vi "input.vi"(8 "error in":errorcluster, 10 "data table in":T1, 11 "JSON_RPC_Interface runtime in":refnum<class "JSON_RPC_Interface runtime.lvclass">) -> (0 "error out":errorcluster, 2 "data table out":T1, 3 "JSON_RPC_Interface runtime out":refnum<class "JSON_RPC_Interface runtime.lvclass">)   [LabVIEW 2017, in "JSON_RPC_Interface runtime.lvclass"]
doc: "Provides an interface for reading data from a module at runtime. While this interface performs no operations, a child should provide an override which may read from any open sessions, references, or interfaces."
uses:
  JSON_RPC_Interface runtime.lvclass
  <vilib>/NI/Tag Bus/table/data table.ctl
  JSON_RPC_Interface runtime.lvclass/JSON_RPC_Interface runtime.ctl
  <vilib>/NI/NI JSONRPC Server Framework/Classes/Request/Request.lvclass/Request.ctl
  <vilib>/NI/Tag Bus/table/data polymorphs/write one/write Double.vi
  <vilib>/NI/Tag Bus/table/data polymorphs/write one/write Single.vi
  <vilib>/NI/Tag Bus/table/data polymorphs/write one/write I64.vi
  <vilib>/NI/Tag Bus/table/data polymorphs/write one/write I32.vi
  <vilib>/NI/Tag Bus/table/data polymorphs/write one/write I16.vi
  <vilib>/NI/Tag Bus/table/data polymorphs/write one/write I8.vi
  <vilib>/NI/Tag Bus/table/data polymorphs/write one/write U64.vi
  <vilib>/NI/Tag Bus/table/data polymorphs/write one/write U32.vi
  <vilib>/NI/Tag Bus/table/data polymorphs/write one/write U16.vi
  <vilib>/NI/Tag Bus/table/data polymorphs/write one/write U8.vi
  <vilib>/NI/Tag Bus/table/data polymorphs/write one/write Array of Double.vi
  <vilib>/NI/Tag Bus/table/data polymorphs/write one/write Array of Single.vi
  <vilib>/NI/Tag Bus/table/data polymorphs/write one/write Array of I32.vi
  <vilib>/NI/Tag Bus/table/data polymorphs/write one/write Array of I16.vi
  <vilib>/NI/Tag Bus/table/data polymorphs/write one/write Array of I8.vi
  <vilib>/NI/Tag Bus/table/data polymorphs/write one/write Array of U64.vi
  <vilib>/NI/Tag Bus/table/data polymorphs/write one/write Array of U32.vi
  <vilib>/NI/Tag Bus/table/data polymorphs/write one/write Array of U16.vi
  <vilib>/NI/Tag Bus/table/data polymorphs/write one/write Array of U8.vi
  <vilib>/NI/Tag Bus/table/data polymorphs/write one/write Array of Boolean.vi
  <vilib>/NI/Tag Bus/table/data polymorphs/write one/write Array of String.vi
  <vilib>/NI/Tag Bus/table/data polymorphs/write one/write Boolean.vi
  <vilib>/NI/Tag Bus/table/data polymorphs/write one/write String.vi
  <vilib>/NI/NI JSONRPC Server Framework/Classes/Request/request.Read params.vi
  <vilib>/NI/NI JSONRPC Server Framework/Classes/Request/request.Read method.vi
  <vilib>/NI/JSON Support for LabVIEW/JSON Value/New JSON Value/New JSON ({String}).vi
  <vilib>/NI/NI JSONRPC Server Framework/Classes/Server/Add Response (Method Not Found from Request).vi
  <vilib>/NI/NI JSONRPC Server Framework/Classes/params/params.To JSON Tree.vi
  <vilib>/NI/NI JSONRPC Server Framework/Classes/Server/Add Response (Invalid Params from Request).vi
  <vilib>/NI/NI JSONRPC Server Framework/Classes/Server/Add Response (Internal Error from Request).vi
  <vilib>/NI/JSON Support for LabVIEW/JSON Value/Object/Insert Value/Insert Value (String).vi
  <vilib>/NI/NI JSONRPC Server Framework/Classes/Server/Add Response (Result from Request).vi
  <vilib>/NI/JSON Support for LabVIEW/JSON Value/JSON Value.lvclass
  <vilib>/NI/NI JSONRPC Server Framework/Classes/Server/JSONRPC Server.lvclass
  <vilib>/NI/Tag Bus/table/data table.lvlib
  <vilib>/NI/NI JSONRPC Server Framework/Classes/Request/Request.lvclass
  <vilib>/NI/JSON Support for LabVIEW/JSON Variant Support/JSON Variant Support.lvclass
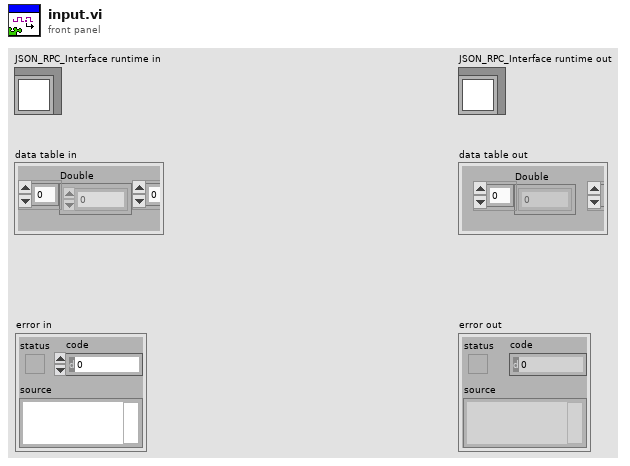
[diagram p1: front panel]
types:
  T1 = typedef "tag bus.lvlib/data table.lvlib/data table.ctl" = cluster{"Double":dbl[], "Single":sgl[], "I64":i64[], "I32":i32[], "I16":i16[], "I8":i8[], "U64":u64[], "U32":u32[], "U16":u16[], "U8":u8[], "Boolean":bool[], "String":string[], "Array of Double":cluster{"DBL Array":dbl[]}[], "Array of Single":cluster{"SGL Array":sgl[]}[], "Array of I64":cluster{"I64 Array":i64[]}[], "Array of I32":cluster{"I32 Array":i32[]}[], "Array of I16":cluster{"I16 Array":i16[]}[], "Array of I8":cluster{"I8 Array":i8[]}[], "Array of U64":cluster{"U64 Array":u64[]}[], "Array of U32":cluster{"U32 Array":u32[]}[], "Array of U16":cluster{"U16 Array":u16[]}[], "Array of U8":cluster{"U8 Array":u8[]}[], "Array of Boolean":cluster{"Boolean Array":bool[]}[], "Array of String":cluster{"String Array":string[]}[]}
  T2 = typedef "tag bus.lvlib/tag descriptor.lvclass/Data Type.ctl" = enum16{"Double", "Single", "I64", "I32", "I16", "I8", "U64", "U32", "U16", "U8", "Boolean", "String", "Array of Double", "Array of Single", "Array of I64", "Array of I32", "Array of I16", "Array of I8", "Array of U64", "Array of U32", "Array of U16", "Array of U8", "Array of Boolean", "Array of String"}
  T3 = cluster{"Numeric":dbl, "Boolean":bool, "String":string, "Array of Numerics":dbl[], "Array of Boolean":bool[], "Array of String":string[]}
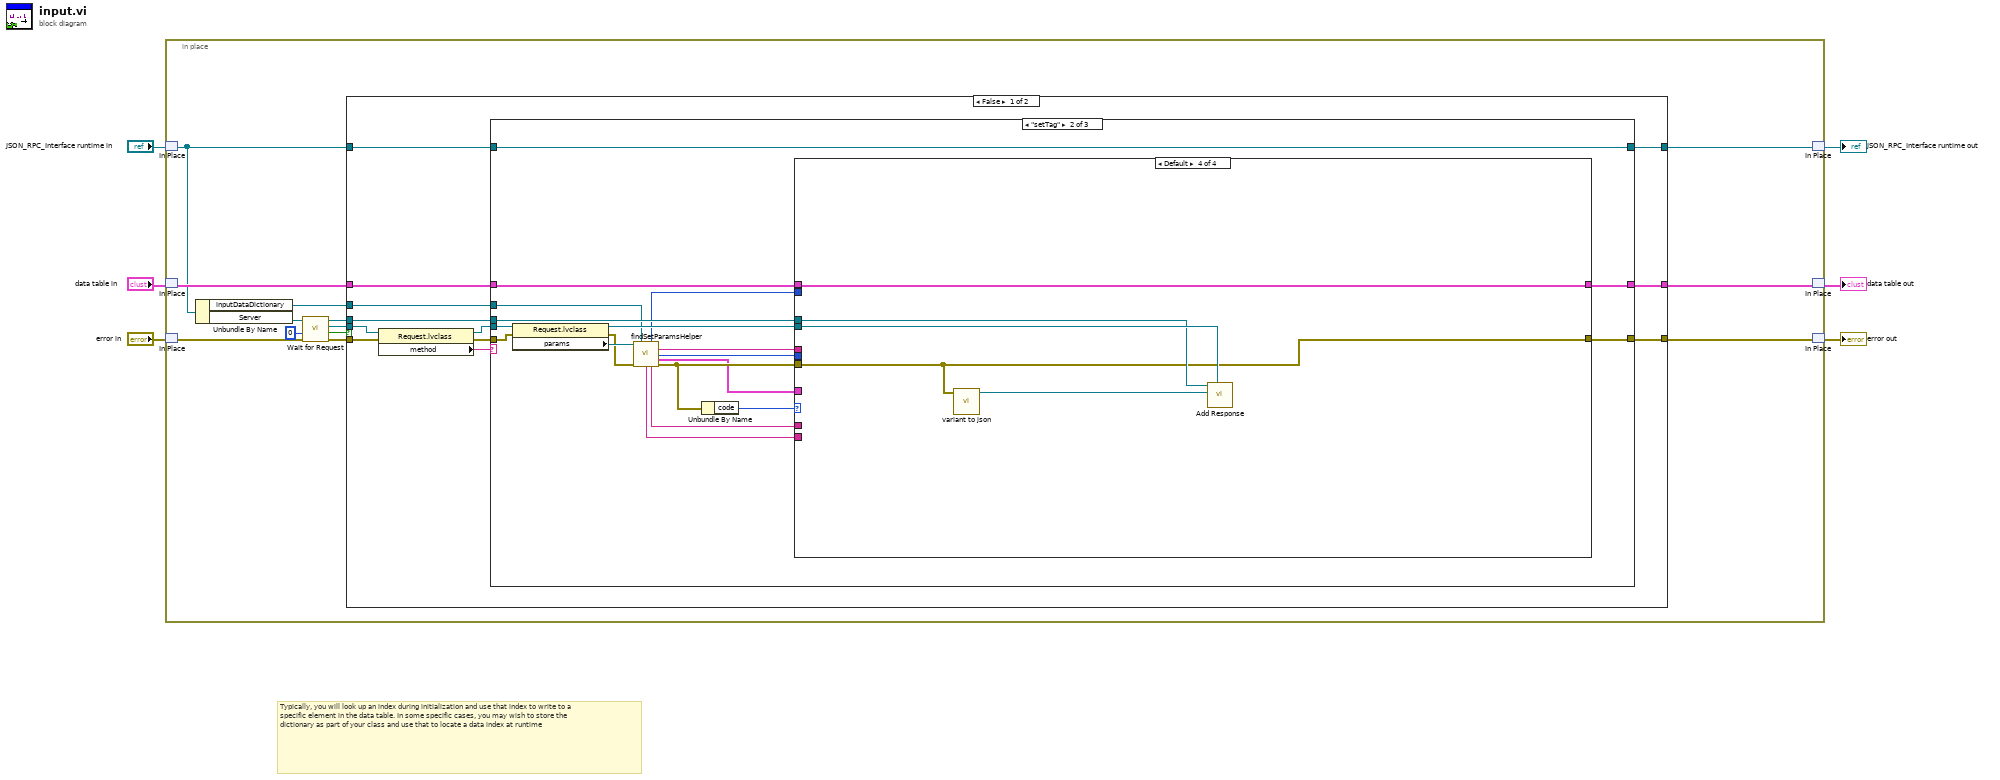
[diagram p0: block diagram]
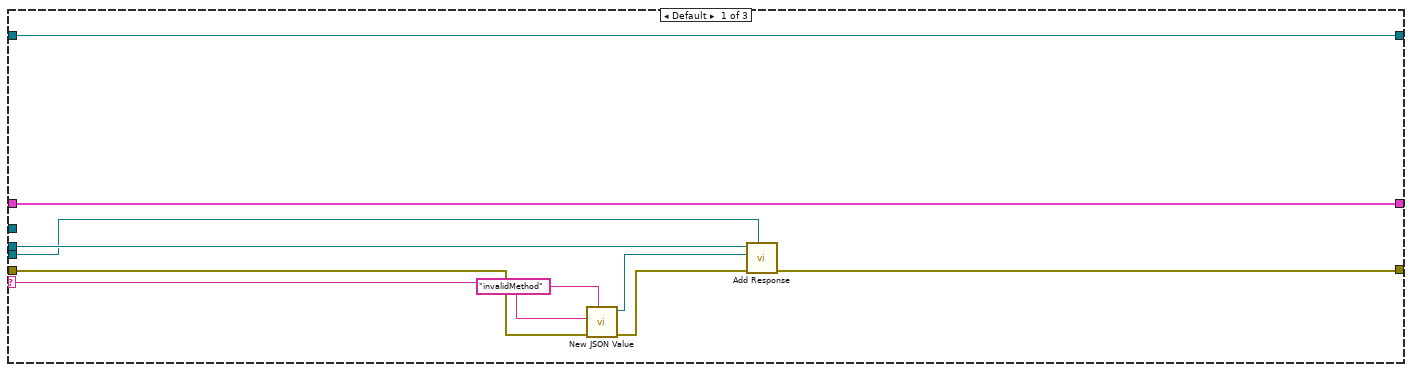
[diagram p2: hidden frame]
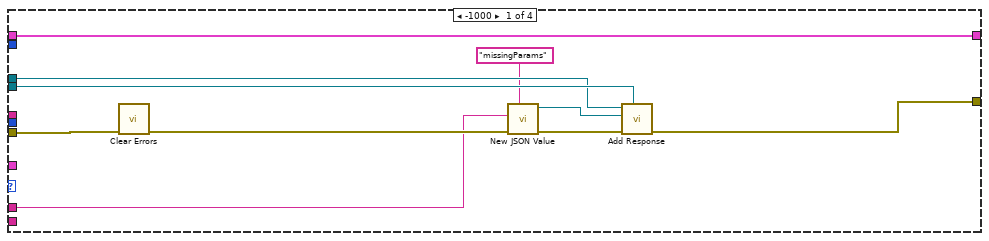
[diagram p3: hidden frame]
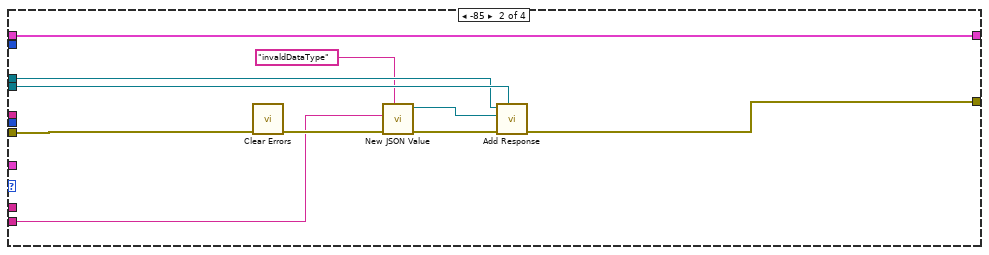
[diagram p4: hidden frame]
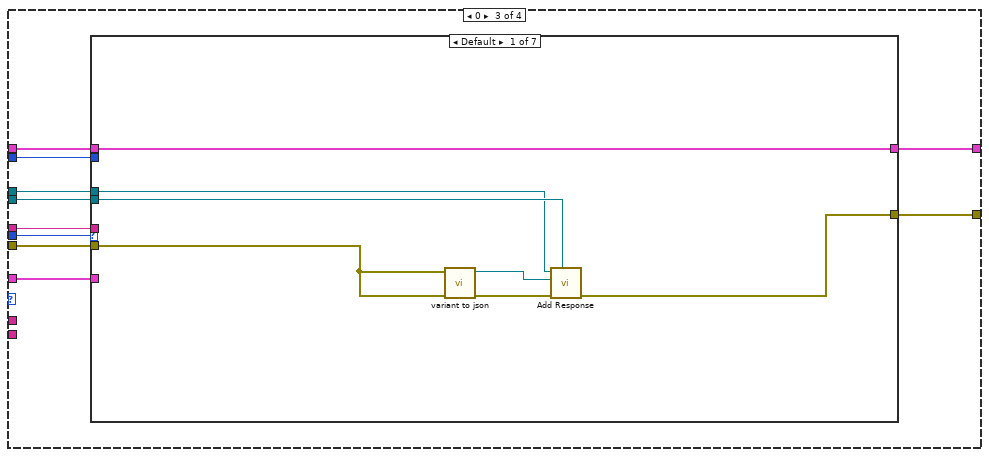
[diagram p5: hidden frame]
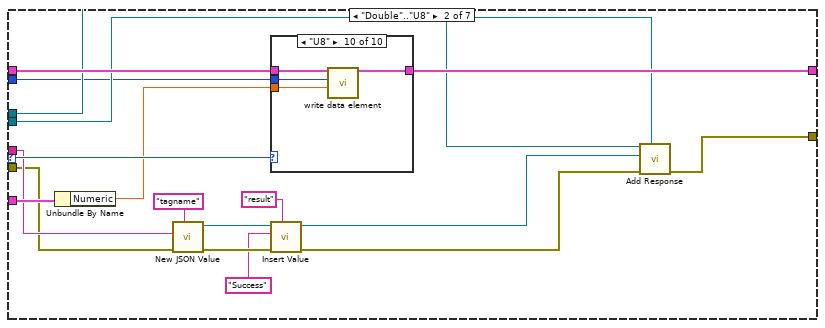
[diagram p6: hidden frame]
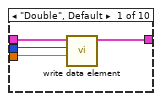
[diagram p7: hidden frame]
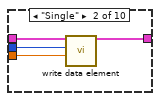
[diagram p8: hidden frame]
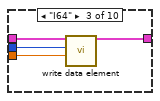
[diagram p9: hidden frame]
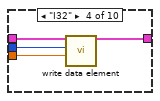
[diagram p10: hidden frame]
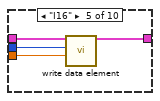
[diagram p11: hidden frame]
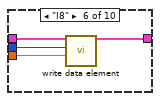
[diagram p12: hidden frame]
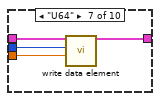
[diagram p13: hidden frame]
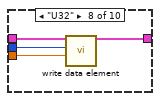
[diagram p14: hidden frame]
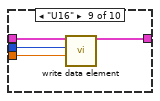
[diagram p15: hidden frame]
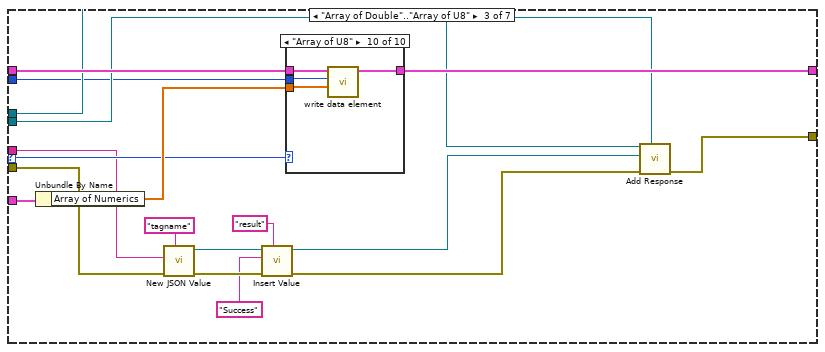
[diagram p16: hidden frame]
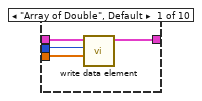
[diagram p17: hidden frame]
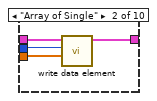
[diagram p18: hidden frame]
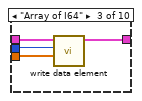
[diagram p19: hidden frame]
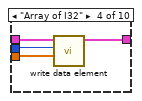
[diagram p20: hidden frame]
diagram:
  # "Typically, you will look up an index during initialization and use that index to write to a specific element in the data table. In some specific cases, you may wish to store the dictionary as part of your class and use that to locate a data index at runtime"
  n1 = in-place {
    n2 = in-place-match #1("JSON_RPC_Interface runtime in") -> (w8:refnum<class "JSON_RPC_Interface runtime.lvclass">)
    n3 = in-place-match #2("data table in") -> (w14:T1)
    n4 = in-place-match #3("error in") -> (w19:errorcluster)
    n5 = Unbundle By Name(w8) -> ("inputDataDictionary"=w9:refnum<class "data dictionary.lvclass">, "Server"=w18:refnum<class "JSONRPC Server.lvclass">)
    n6 = call <vilib>:"Wait for Request.vi"("error in (no error)"=w19, "timeout in ms (100)"=0, "Server in"=w18) -> ("error out"=w15:errorcluster, "timed out?"=w11:bool, "Request"=w16:refnum<class "Request.lvclass">, "Server out"=w10:refnum<class "JSONRPC Server.lvclass">)  [unwired: 5 in]
    n7 = case shown="False" w11 {
      tunnel: w16 -> [w31 _]
      tunnel: w15 -> [w30 w294]
      tunnel: w14 -> [w28 w295]
      tunnel: [w25 w295] -> w13
      tunnel: [w24 w294] -> w12
      tunnel: w10 -> [w23 _]
      tunnel: w9 -> [w22 _]
      tunnel: w8 -> [w21 w293]
      tunnel: [w20 w293] -> w7
      frame False {
        n8 = property class="Request.lvclass"(reference=w31, error in=w30) -> (reference out=w27:refnum<class "Request.lvclass">, error out=w26:errorcluster, "method"=w29:string)
        n9 = case shown="\"setTag\"" w29 {
          selector: w29 -> [w38 _ _]
          tunnel: w28 -> [w33 w58 w290]
          tunnel: w27 -> [w39 w60 w288]
          tunnel: w26 -> [w35 w59 w289]
          tunnel: [w33 w57 w290] -> w25
          tunnel: [w40 w53 w289] -> w24
          tunnel: w23 -> [w41 w56 _]
          tunnel: w22 -> [_ w43 _]
          tunnel: w21 -> [w32 w52 w292]
          tunnel: [w32 w52 w291] -> w20
          frame Default {
            n10 = call-poly <vilib>:"New JSON Value.vi"("key"="invalidMethod", "error in (no error)"=w35, "value"=w38) -> ("error out"=w34:errorcluster, "JSON Value out"=w37:refnum<class "JSON Value.lvclass">)  [unwired: 7 in]
            n11 = call-poly <vilib>:"Add Response.vi"("Request"=w39, "error in (no error)"=w34, "data"=w37, "Server in"=w41) -> ("error out"=w40:errorcluster)  [unwired: 5 in, 2 out]
          }
          frame "setTag" {
            n12 = property class="Request.lvclass"(reference=w60, error in=w59) -> (reference out=w54:refnum<class "Request.lvclass">, error out=w50:errorcluster, "params"=w51:refnum<class "JSON Value.lvclass">)
            n13 = call "findSetParamsHelper.vi"("params in"=w51, "inputDataDictionary"=w43, "error in"=w50) -> ("tagindex"=w42:i32, "tagname"=w48:string, "tagtype"=w47:T2, "tagdata"=w44:T3, "invalidTagType"=w45:string, "missingParam"=w46:string, "error out"=w49:errorcluster)  [unwired: 5 in, 1 out]
            n14 = Unbundle By Name(w49) -> ("code"=w55:i32)
            n15 = case shown="Default" w55 {
              tunnel: w49 -> [w65 w77 w82 w283]
              tunnel: w58 -> [w62 w75 w90 w286]
              tunnel: w48 -> [_ _ w89 _]
              tunnel: [w62 w75 w88 w286] -> w57
              tunnel: w56 -> [w69 w73 w87 w284]
              tunnel: w54 -> [w70 w74 w86 w285]
              tunnel: [w63 w76 w85 w283] -> w53
              tunnel: w47 -> [_ _ w84 _]
              tunnel: w44 -> [_ _ w83 _]
              tunnel: w46 -> [w61 _ _ _]
              tunnel: w45 -> [_ w71 _ _]
              tunnel: w42 -> [_ _ w81 _]
              frame -1000 {
                n16 = call <vilib>:"Clear Errors.vi"("error in (no error)"=w65) -> ("error out"=w64:errorcluster)  [unwired: 5 in, 1 out]
                n17 = call-poly <vilib>:"New JSON Value.vi"("key"="missingParams", "error in (no error)"=w64, "value"=w61) -> ("error out"=w67:errorcluster, "JSON Value out"=w66:refnum<class "JSON Value.lvclass">)  [unwired: 7 in]
                n18 = call-poly <vilib>:"Add Response.vi"("Request"=w70, "error in (no error)"=w67, "data"=w66, "Server in"=w69) -> ("error out"=w63:errorcluster)  [unwired: 5 in, 2 out]
              }
              frame -85 {
                n19 = call <vilib>:"Clear Errors.vi"("error in (no error)"=w77) -> ("error out"=w78:errorcluster)  [unwired: 5 in, 1 out]
                n20 = call-poly <vilib>:"New JSON Value.vi"("key"="invaldDataType", "error in (no error)"=w78, "value"=w71) -> ("error out"=w80:errorcluster, "JSON Value out"=w79:refnum<class "JSON Value.lvclass">)  [unwired: 7 in]
                n21 = call-poly <vilib>:"Add Response.vi"("Request"=w74, "error in (no error)"=w80, "data"=w79, "Server in"=w73) -> ("error out"=w76:errorcluster)  [unwired: 5 in, 2 out]
              }
              frame 0 {
                n22 = case shown="Default" w84 {
                  selector: w84 -> [_ w109 w165 _ _ _ _]
                  tunnel: w89 -> [_ w105 w159 w217 w231 w251 w268]
                  tunnel: w90 -> [w97 w115 w173 w230 w247 w264 w281]
                  tunnel: [w97 w114 w172 w229 w246 w263 w280] -> w88
                  tunnel: w87 -> [w95 w111 w169 w226 w243 w260 w277]
                  tunnel: w82 -> [w91 w104 w158 w216 w234 w250 w267]
                  tunnel: w86 -> [w96 w112 w170 w227 w244 w261 w278]
                  tunnel: [w94 w113 w171 w228 w245 w262 w279] -> w85
                  tunnel: w83 -> [_ w108 w167 w224 w241 w258 w275]
                  tunnel: w81 -> [_ w110 w168 w225 w242 w259 w276]
                  frame Default {
                    n23 = call <vilib>:"variant to json.vi"("error in (no error)"=w91, "Variant"=w91) -> ("error out"=w93:errorcluster, "JSON Value"=w92:refnum<class "JSON Value.lvclass">)  [unwired: 8 in]
                    n24 = call-poly <vilib>:"Add Response.vi"("Request"=w96, "error in (no error)"=w93, "data"=w92, "Server in"=w95) -> ("error out"=w94:errorcluster)  [unwired: 5 in, 2 out]
                  }
                  frame "Double".."U8" {
                    n25 = Unbundle By Name(w108) -> ("Numeric"=w107:dbl)
                    n26 = call-poly <vilib>:"New JSON Value.vi"("key"="tagname", "error in (no error)"=w104, "value"=w105) -> ("error out"=w102:errorcluster, "JSON Value out"=w103:refnum<class "JSON Value.lvclass">)  [unwired: 7 in]
                    n27 = case shown="\"U8\"" w109 {
                      tunnel: w115 -> [w119 w123 w127 w131 w135 w139 w143 w147 w151 w155]
                      tunnel: [w118 w122 w126 w130 w134 w138 w142 w146 w150 w154] -> w114
                      tunnel: w110 -> [w116 w121 w125 w129 w133 w137 w141 w145 w149 w153]
                      tunnel: w107 -> [w117 w120 w124 w128 w132 w136 w140 w144 w148 w152]
                      frame "Double", Default {
                        n28 = call-poly <vilib>:"write data element.vi"("value"=w117, "index"=w116, "data table in"=w119) -> ("data table out"=w118:T1)  [unwired: 8 in]
                      }
                      frame "Single" {
                        n29 = call-poly <vilib>:"write data element.vi"("value"=w120, "index"=w121, "data table in"=w123) -> ("data table out"=w122:T1)  [unwired: 8 in]
                      }
                      frame "I64" {
                        n30 = call-poly <vilib>:"write data element.vi"("value"=w124, "index"=w125, "data table in"=w127) -> ("data table out"=w126:T1)  [unwired: 8 in]
                      }
                      frame "I32" {
                        n31 = call-poly <vilib>:"write data element.vi"("value"=w128, "index"=w129, "data table in"=w131) -> ("data table out"=w130:T1)  [unwired: 8 in]
                      }
                      frame "I16" {
                        n32 = call-poly <vilib>:"write data element.vi"("value"=w132, "index"=w133, "data table in"=w135) -> ("data table out"=w134:T1)  [unwired: 8 in]
                      }
                      frame "I8" {
                        n33 = call-poly <vilib>:"write data element.vi"("value"=w136, "index"=w137, "data table in"=w139) -> ("data table out"=w138:T1)  [unwired: 8 in]
                      }
                      frame "U64" {
                        n34 = call-poly <vilib>:"write data element.vi"("value"=w140, "index"=w141, "data table in"=w143) -> ("data table out"=w142:T1)  [unwired: 8 in]
                      }
                      frame "U32" {
                        n35 = call-poly <vilib>:"write data element.vi"("value"=w144, "index"=w145, "data table in"=w147) -> ("data table out"=w146:T1)  [unwired: 8 in]
                      }
                      frame "U16" {
                        n36 = call-poly <vilib>:"write data element.vi"("value"=w148, "index"=w149, "data table in"=w151) -> ("data table out"=w150:T1)  [unwired: 8 in]
                      }
                      frame "U8" {
                        n37 = call-poly <vilib>:"write data element.vi"("value"=w152, "index"=w153, "data table in"=w155) -> ("data table out"=w154:T1)  [unwired: 8 in]
                      }
                    }
                    n38 = call-poly <vilib>:"Insert Value.vi"("key"="result", "error in (no error)"=w102, "value"="Success" ("key"), "JSON Value in"=w103) -> ("error out"=w98:errorcluster, "JSON Value out"=w99:refnum<class "JSON Value.lvclass">)  [unwired: 5 in, 1 out]
                    n39 = call-poly <vilib>:"Add Response.vi"("Request"=w112, "error in (no error)"=w98, "JSON Value in"=w99, "Server in"=w111) -> ("error out"=w113:errorcluster)  [unwired: 5 in, 2 out]
                  }
                  frame "Array of Double".."Array of U8" {
                    n40 = Unbundle By Name(w167) -> ("Array of Numerics"=w166:dbl[])
                    n41 = call-poly <vilib>:"New JSON Value.vi"("key"="tagname", "error in (no error)"=w158, "value"=w159) -> ("error out"=w162:errorcluster, "JSON Value out"=w163:refnum<class "JSON Value.lvclass">)  [unwired: 7 in]
                    n42 = call-poly <vilib>:"Insert Value.vi"("key"="result", "error in (no error)"=w162, "value"="Success" ("key"), "JSON Value in"=w163) -> ("error out"=w156:errorcluster, "JSON Value out"=w157:refnum<class "JSON Value.lvclass">)  [unwired: 5 in, 1 out]
                    n43 = case shown="\"Array of U8\"" w165 {
                      tunnel: w173 -> [w177 w181 w185 w189 w193 w197 w201 w205 w209 w213]
                      tunnel: [w176 w180 w184 w188 w192 w196 w200 w204 w208 w212] -> w172
                      tunnel: w168 -> [w174 w178 w182 w186 w190 w194 w198 w202 w206 w210]
                      tunnel: w166 -> [w175 w179 w183 w187 w191 w195 w199 w203 w207 w211]
                      frame "Array of Double", Default {
                        n44 = call-poly <vilib>:"write data element.vi"("value"=w175, "index"=w174, "data table in"=w177) -> ("data table out"=w176:T1)  [unwired: 8 in]
                      }
                      frame "Array of Single" {
                        n45 = call-poly <vilib>:"write data element.vi"("value"=w179, "index"=w178, "data table in"=w181) -> ("data table out"=w180:T1)  [unwired: 8 in]
                      }
                      frame "Array of I64" {
                        n46 = call-poly <vilib>:"write data element.vi"("value"=w183, "index"=w182, "data table in"=w185) -> ("data table out"=w184:T1)  [unwired: 8 in]
                      }
                      frame "Array of I32" {
                        n47 = call-poly <vilib>:"write data element.vi"("value"=w187, "index"=w186, "data table in"=w189) -> ("data table out"=w188:T1)  [unwired: 8 in]
                      }
                      frame "Array of I16" {
                        n48 = call-poly <vilib>:"write data element.vi"("value"=w191, "index"=w190, "data table in"=w193) -> ("data table out"=w192:T1)  [unwired: 8 in]
                      }
                      frame "Array of I8" {
                        n49 = call-poly <vilib>:"write data element.vi"("value"=w195, "index"=w194, "data table in"=w197) -> ("data table out"=w196:T1)  [unwired: 8 in]
                      }
                      frame "Array of U64" {
                        n50 = call-poly <vilib>:"write data element.vi"("value"=w199, "index"=w198, "data table in"=w201) -> ("data table out"=w200:T1)  [unwired: 8 in]
                      }
                      frame "Array of U32" {
                        n51 = call-poly <vilib>:"write data element.vi"("value"=w203, "index"=w202, "data table in"=w205) -> ("data table out"=w204:T1)  [unwired: 8 in]
                      }
                      frame "Array of U16" {
                        n52 = call-poly <vilib>:"write data element.vi"("value"=w207, "index"=w206, "data table in"=w209) -> ("data table out"=w208:T1)  [unwired: 8 in]
                      }
                      frame "Array of U8" {
                        n53 = call-poly <vilib>:"write data element.vi"("value"=w211, "index"=w210, "data table in"=w213) -> ("data table out"=w212:T1)  [unwired: 8 in]
                      }
                    }
                    n54 = call-poly <vilib>:"Add Response.vi"("Request"=w170, "error in (no error)"=w156, "JSON Value in"=w157, "Server in"=w169) -> ("error out"=w171:errorcluster)  [unwired: 5 in, 2 out]
                  }
                  frame "Array of Boolean" {
                    n55 = Unbundle By Name(w224) -> ("Array of Boolean"=w223:bool[])
                    n56 = call-poly <vilib>:"New JSON Value.vi"("key"="tagname", "error in (no error)"=w216, "value"=w217) -> ("error out"=w220:errorcluster, "JSON Value out"=w221:refnum<class "JSON Value.lvclass">)  [unwired: 7 in]
                    n57 = call-poly <vilib>:"write data element.vi"("value"=w223, "index"=w225, "data table in"=w230) -> ("data table out"=w229:T1)  [unwired: 8 in]
                    n58 = call-poly <vilib>:"Insert Value.vi"("key"="result", "error in (no error)"=w220, "value"="Success" ("key"), "JSON Value in"=w221) -> ("error out"=w214:errorcluster, "JSON Value out"=w215:refnum<class "JSON Value.lvclass">)  [unwired: 5 in, 1 out]
                    n59 = call-poly <vilib>:"Add Response.vi"("Request"=w227, "error in (no error)"=w214, "JSON Value in"=w215, "Server in"=w226) -> ("error out"=w228:errorcluster)  [unwired: 5 in, 2 out]
                  }
                  frame "Array of String" {
                    n60 = Unbundle By Name(w241) -> ("Array of String"=w240:string[])
                    n61 = call-poly <vilib>:"New JSON Value.vi"("key"="tagname", "error in (no error)"=w234, "value"=w231) -> ("error out"=w237:errorcluster, "JSON Value out"=w238:refnum<class "JSON Value.lvclass">)  [unwired: 7 in]
                    n62 = call-poly <vilib>:"write data element.vi"("value"=w240, "index"=w242, "data table in"=w247) -> ("data table out"=w246:T1)  [unwired: 8 in]
                    n63 = call-poly <vilib>:"Insert Value.vi"("key"="result", "error in (no error)"=w237, "value"="Success" ("key"), "JSON Value in"=w238) -> ("error out"=w233:errorcluster, "JSON Value out"=w232:refnum<class "JSON Value.lvclass">)  [unwired: 5 in, 1 out]
                    n64 = call-poly <vilib>:"Add Response.vi"("Request"=w244, "error in (no error)"=w233, "JSON Value in"=w232, "Server in"=w243) -> ("error out"=w245:errorcluster)  [unwired: 5 in, 2 out]
                  }
                  frame "Boolean" {
                    n65 = Unbundle By Name(w258) -> ("Boolean"=w257:bool)
                    n66 = call-poly <vilib>:"New JSON Value.vi"("key"="tagname", "error in (no error)"=w250, "value"=w251) -> ("error out"=w254:errorcluster, "JSON Value out"=w255:refnum<class "JSON Value.lvclass">)  [unwired: 7 in]
                    n67 = call-poly <vilib>:"write data element.vi"("value"=w257, "index"=w259, "data table in"=w264) -> ("data table out"=w263:T1)  [unwired: 8 in]
                    n68 = call-poly <vilib>:"Insert Value.vi"("key"="result", "error in (no error)"=w254, "value"="Success" ("key"), "JSON Value in"=w255) -> ("error out"=w249:errorcluster, "JSON Value out"=w248:refnum<class "JSON Value.lvclass">)  [unwired: 5 in, 1 out]
                    n69 = call-poly <vilib>:"Add Response.vi"("Request"=w261, "error in (no error)"=w249, "JSON Value in"=w248, "Server in"=w260) -> ("error out"=w262:errorcluster)  [unwired: 5 in, 2 out]
                  }
                  frame "String" {
                    n70 = Unbundle By Name(w275) -> ("String"=w274:string)
                    n71 = call-poly <vilib>:"New JSON Value.vi"("key"="tagname", "error in (no error)"=w267, "value"=w268) -> ("error out"=w271:errorcluster, "JSON Value out"=w272:refnum<class "JSON Value.lvclass">)  [unwired: 7 in]
                    n72 = call-poly <vilib>:"write data element.vi"("value"=w274, "index"=w276, "data table in"=w281) -> ("data table out"=w280:T1)  [unwired: 8 in]
                    n73 = call-poly <vilib>:"Insert Value.vi"("key"="result", "error in (no error)"=w271, "value"="Success" ("key"), "JSON Value in"=w272) -> ("error out"=w266:errorcluster, "JSON Value out"=w265:refnum<class "JSON Value.lvclass">)  [unwired: 5 in, 1 out]
                    n74 = call-poly <vilib>:"Add Response.vi"("Request"=w278, "error in (no error)"=w266, "JSON Value in"=w265, "Server in"=w277) -> ("error out"=w279:errorcluster)  [unwired: 5 in, 2 out]
                  }
                }
              }
              frame Default {
                n75 = call <vilib>:"variant to json.vi"("Variant"=w283) -> ("JSON Value"=w282:refnum<class "JSON Value.lvclass">)  [unwired: 9 in, 1 out]
                n76 = call-poly <vilib>:"Add Response.vi"("Request"=w285, "data"=w282, "Server in"=w284) -> ()  [unwired: 6 in, 3 out]
              }
            }
          }
          frame "getTag" {
            n77 = Bundle By Name(cluster=w292, "getTagRequest"=w288, "getTagFlag"=TRUE) -> (w291:refnum<class "JSON_RPC_Interface runtime.lvclass">)
          }
        }
      }
      frame True {
      }
    }
    n78 = in-place-match #1(w7) -> (→"JSON_RPC_Interface runtime out":refnum<class "JSON_RPC_Interface runtime.lvclass">)
    n79 = in-place-match #2(w13) -> (→"data table out":T1)
    n80 = in-place-match #3(w12) -> (→"error out":errorcluster)
  }
